vi "VDH-calibrateS11.vi"(7 "Calibration Factor":T1, 10 "S11":cdb[](array[numeric])) -> (2 "S11 out":cdb[](array[numeric]))   [LabVIEW 2020, in "VDH-VNA_data_handler.lvlib" / "VDH-VNA_data_handler.lvclass"]
uses:
  VDH-VNA_data_handler.lvclass
  VDH-Calibration_factor.ctl
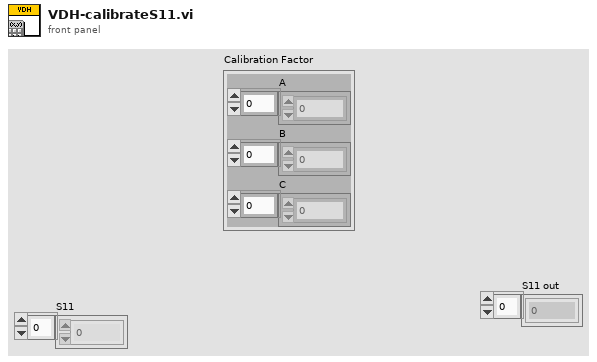
[diagram p1: front panel]
types:
  T1 = typedef "VDH-VNA_data_handler.lvlib/VDH-VNA_data_handler.lvclass/VDH-Calibration_factor.ctl" = cluster{"A":cdb[], "B":cdb[], "C":cdb[]}
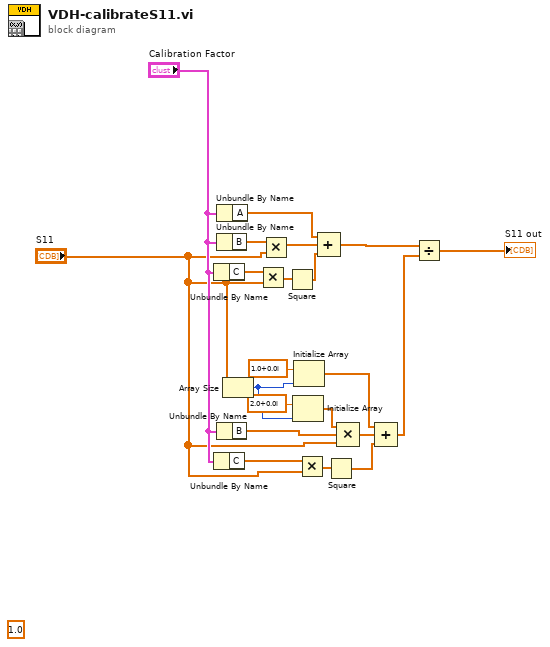
[diagram p0: block diagram]
diagram:
  (unwired) 1.0
  n1 = Unbundle By Name("Calibration Factor") -> ("C"=w21:cdb[])
  n2 = Unbundle By Name("Calibration Factor") -> ("C"=w12:cdb[])
  n3 = Unbundle By Name("Calibration Factor") -> ("A"=w16:cdb[])
  n4 = Unbundle By Name("Calibration Factor") -> ("B"=w19:cdb[])
  n5 = Unbundle By Name("Calibration Factor") -> ("B"=w6:cdb[])
  n6 = Array Size(array="S11") -> (size(s)=w4:i32)
  n7 = Multiply(x=w21, y="S11") -> (x*y=w20:cdb[])
  n8 = Multiply(x=w19, y="S11") -> (x*y=w17:cdb[])
  n9 = Square(x=w20) -> (x^2=w18:cdb[])
  n10 = Initialize Array(cdb 2.0+0.0i, w4) -> (w5:cdb[])
  n11 = Initialize Array(cdb 1.0+0.0i, w4) -> (w9:cdb[])
  n12 = Multiply(x=w12, y="S11") -> (x*y=w13:cdb[])
  n13 = Compound Arithmetic op=ADD(w16, w17, w18) -> (w15:cdb[])
  n14 = Square(x=w13) -> (x^2=w14:cdb[])
  n15 = Compound Arithmetic op=MULTIPLY(w5, w6, "S11") -> (w2:cdb[])
  n16 = Compound Arithmetic op=ADD(w9, w2, w14) -> (w8:cdb[])
  n17 = Divide(x=w15, y=w8) -> (x/y=→"S11 out":cdb[])
